vi "Draw_Box.vi"(8 "Error":errorcluster, 9 "Box Data":T1={"Region"={"Left"=0, "Top"=0, "Right"=0, "Bottom"=0, "Width"=0, "Height"=0, "Start"={"Left"=0, "Top"=0}}, "Color"=0, "Fill?"=TRUE}, 11 "ICON":T4 caption="Icon") -> (0 "Error Out":errorcluster, 3 "ICON Out":T4 caption="Icon")   [LabVIEW 2009]
doc: "Draw a box in the icon"
uses:
  Controls/String_Picture/Picture_Icon.ctl
  Controls/Cluster/Cluster_BOX Data.ctl
  Controls/Cluster/Cluster_Region info.ctl
  Controls/Cluster/Cluster_Top Left position.ctl
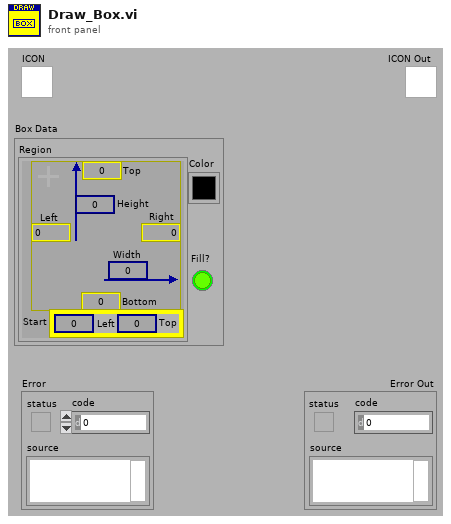
[diagram p1: front panel]
types:
  T1 = typedef "Cluster_BOX Data.ctl" = cluster{"Region":T2, "Color":u32, "Fill?":bool}
  T2 = typedef "Cluster_Region info.ctl" = cluster{"Left":i32, "Top":i32, "Right":i32, "Bottom":i32, "Width":u32, "Height":u32, "Start":T3}
  T3 = typedef "Cluster_Top Left position.ctl" = cluster{"Left":i32, "Top":i32}
  T4 = typedef "Picture_Icon.ctl" = picture
  T5 = cluster{"left":i16, "top":i16, "right":i16, "bottom":i16}
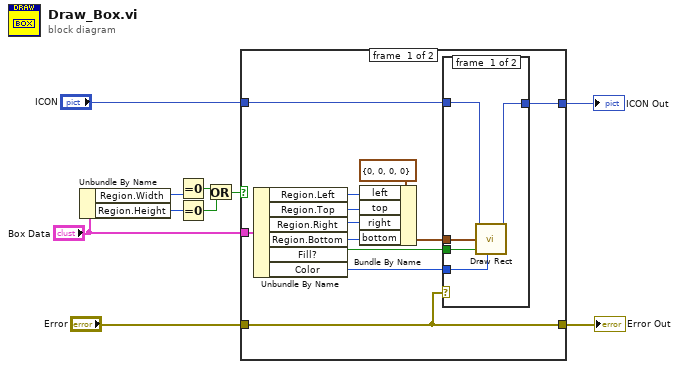
[diagram p0: block diagram]
diagram:
  n1 = Unbundle By Name("Box Data") -> ("Region.Width"=w3:u32, "Region.Height"=w4:u32)
  n2 = Equal To 0?(x=w3) -> (x = 0?=w6:bool)
  n3 = Equal To 0?(x=w4) -> (x = 0?=w7:bool)
  n4 = Or(x=w6, y=w7) -> (x .or. y?=w2:bool)
  n5 = case shown="False" w2 {
    tunnel: "ICON" -> [w22 w30]
    tunnel: [w21 w30] -> w9
    tunnel: "Error" -> [w11 w29]
    tunnel: "Box Data" -> [w12 _]
    tunnel: [w11 w29] -> w1
    frame #0 {
      n6 = Unbundle By Name(w12) -> ("Region.Left"=w17:i32, "Region.Top"=w16:i32, "Region.Right"=w15:i32, "Region.Bottom"=w14:i32, "Fill?"=w20:bool, "Color"=w19:u32)
      n7 = Bundle By Name(cluster=T5 {"left"=0, "top"=0, "right"=0, "bottom"=0} ("rect"), "left"=w17, "top"=w16, "right"=w15, "bottom"=w14) -> (w13:T5)
      n8 = case shown="No Error" w11 {
        tunnel: w19 -> [w27 _]
        tunnel: w22 -> [w26 w28]
        tunnel: w20 -> [w25 _]
        tunnel: [w24 w28] -> w21
        tunnel: w13 -> [w23 _]
        frame #0 {
          n9 = call <vilib>:"Draw Rect.vi"("picture"=w26, "rect"=w23, "fill?(F)"=w25, "color(black)"=w27) -> ("new picture"=w24:picture)  [unwired: 5 in]
        }
        frame #1 {
        }
      }
    }
    frame #1 {
    }
  }
  "Error Out" <- w1
  "ICON Out" <- w9
